vi "makeTrialList (SubVI).vi"(5 "Protocol in":T1={"Subject ID"=enum."S000", "1st Handle Left?"=FALSE, "Trial #"=0, "unit"=enum."IL", "unit #"=0, "Trial list"=[], "count in unit"=0, "IL count"=19, "PT count"=3, "postL sessions"=19, "TR max count"=1} {"TR max count" min=1 max=3 step=1; "postL sessions" min=1 max=100 step=1; "PT count" min=1 max=3 step=1}) -> (0 "Unit Trial count":i32[](array[numeric]), 1 "total trial count":i32, 2 "Protocol out":T1={"Subject ID"=enum."S000", "1st Handle Left?"=FALSE, "Trial #"=0, "unit"=enum."IL", "unit #"=0, "Trial list"=[16, 1, 3, 3, 3, 1, 3, 1, 3, 2, 3, 1, 3, 3, 3, 3, 3, 2, 3, 2, 3, 2, 3, 3, 3, 3, 3, 1, 3, 3, 3, 2, 3], "count in unit"=0, "IL count"=19, "PT count"=3, "postL sessions"=16, "TR max count"=3} {"TR max count" min=1 max=3 step=1; "postL sessions" min=1 max=100 step=1; "PT count" min=1 max=3 step=1})   [LabVIEW 2011]
uses:
  ctlProtocol.ctl
  ctlProtocolSubID.ctl
  ctlProtocolUnit.ctl
  <vilib>/Analysis/1siggen.llb/Riffle Array (I32).vi
  <vilib>/Analysis/NI_AALBase.lvlib
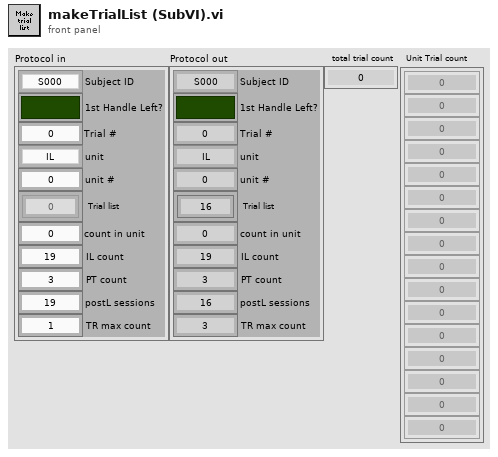
[diagram p1: front panel]
types:
  T1 = typedef "ctlProtocol.ctl" = cluster{"Subject ID":T2, "1st Handle Left?":bool, "Trial #":i32, "unit":T3, "unit #":i32, "Trial list":i32[], "count in unit":i32, "IL count":i32, "PT count":i32, "postL sessions":i32, "TR max count":i32}
  T2 = typedef "ctlProtocolSubID.ctl" = enum16{"S000", "S001", "S002", "S003", "S004", "S005", "S006", "S007", "S008", "S009", "S010", "S011", "S012", "S013", "S014", "S015", "S016", "S017", "S018", "S019", "S020", "S021", "S022", "S023", "S024", "S025", "S026", "S027", "S028", "S029", "S030"}
  T3 = typedef "ctlProtocolUnit.ctl" = enum16{"IL", "TR", "PT"}
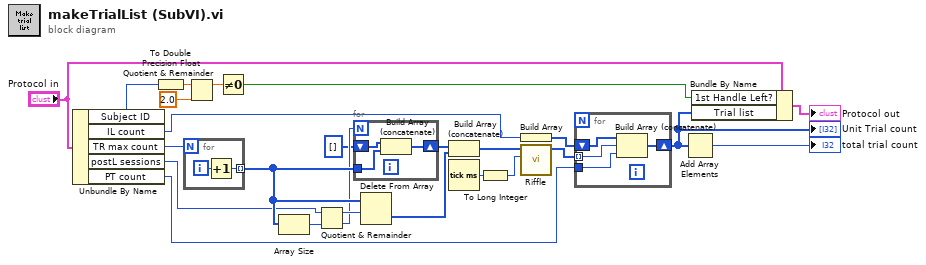
[diagram p0: block diagram]
diagram:
  n1 = Unbundle By Name("Protocol in") -> ("Subject ID"=w5:T2, "IL count"=w13:i32, "TR max count"=w12:i32, "postL sessions"=w11:i32, "PT count"=w10:i32)
  n2 = To Double Precision Float(number=w5) -> (double precision float=w4:dbl)
  n3 = for {
    N: w12 -> [_]
    tunnel: [w26] -> w25 mode=indexing
    i -> [w27]
    n4 = Increment(x=w27) -> (x+1=w26:i32)
  }
  n5 = Quotient & Remainder(x=w4, y=2.0) -> (x-y*floor(x/y)=w2:dbl)  [unwired: 1 out]
  n6 = Not Equal To 0?(x=w2) -> (x != 0?=w1:bool)
  n7 = Array Size(array=w25) -> (size(s)=w22:i32)
  n8 = Quotient & Remainder(x=w11, y=w22) -> (x-y*floor(x/y)=w23:i32, floor(x/y)=w21:i32)
  n9 = for {
    N: w21 -> [_]
    shift-right: [w30] -> w15
    shift-left: i32[] [] -> [w29]
    tunnel: w25 -> [w28]
    n10 = Build Array (concatenate)(w29, w28) -> (w30:i32[])
  }
  n11 = Delete From Array(array=w25, length=w23) -> (deleted portion=w24:i32[])  [unwired: 1 in, 1 out]
  n12 = Build Array (concatenate)(w15, w24) -> (w16:i32[])
  n13 = Tick Count (ms)() -> (millisecond timer value=w17:u32)
  n14 = To Long Integer(number=w17) -> (32bit integer=w18:i32)
  n15 = Build Array(w13) -> (w20:i32[])
  n16 = call-poly <vilib>:"Riffle.vi"("seed"=w18, "X"=w16) -> ("Riffled {X}"=w19:i32[])  [unwired: 7 in, 2 out]
  n17 = for {
    tunnel: w19 -> [w34] mode=indexing
    shift-right: [w33] -> w6
    shift-left: w20 -> [w32]
    tunnel: w10 -> [w31]
    n18 = Build Array (concatenate)(w32, w34, w31) -> (w33:i32[])
  }
  "Unit Trial count" <- w6
  n19 = Add Array Elements(numeric array=w6) -> (sum=→"total trial count":i32)
  n20 = Bundle By Name(cluster="Protocol in", "1st Handle Left?"=w1, "Trial list"=w6) -> (→"Protocol out":T1)
